vi "set transfer settings id.vi"(8 "error in (no error)":errorcluster, 9 "settings id":string, 10 "id":string, 11 "DSFConfiguration in":refnum<class "DSFConfiguration.lvclass">) -> (0 "error out":errorcluster, 3 "DSFConfiguration out":refnum<class "DSFConfiguration.lvclass">)   [LabVIEW 2017, in "DSFConfiguration.lvclass"]
uses:
  DSFConfiguration.lvclass
  DSFConfiguration.lvclass/DSFConfiguration.ctl
  DSFTransfer/DSFTransfer.lvclass/DSFTransfer.ctl
  DSFTransfer/Write settings id.vi
  DSFTransfer/DSFTransfer.lvclass
  C:/github/data-sharing-framework/Source/Configuration API/Classes/IDable/IDable.lvclass
  DSFPluginSettings/DSFPluginSettings.lvclass
  ID API/ID API.lvclass
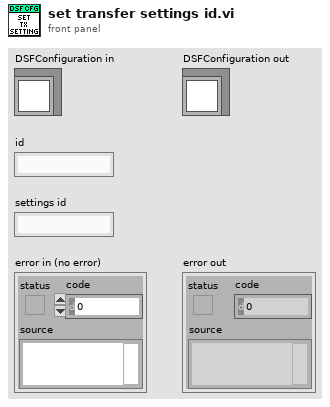
[diagram p1: front panel]
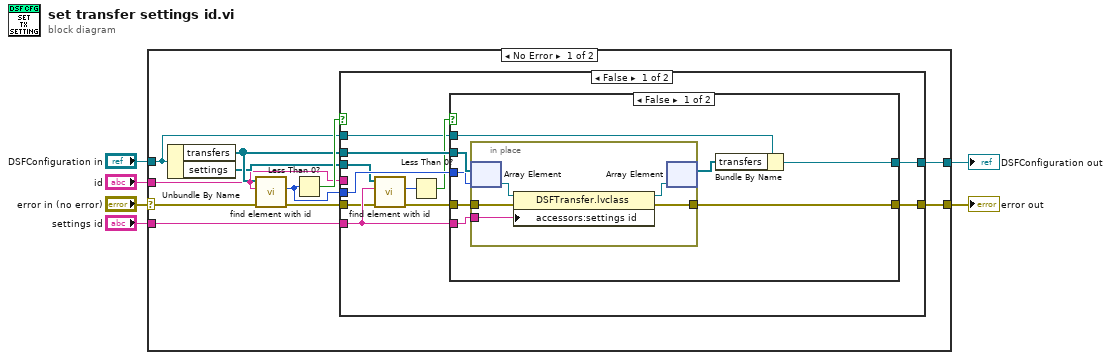
[diagram p0: block diagram]
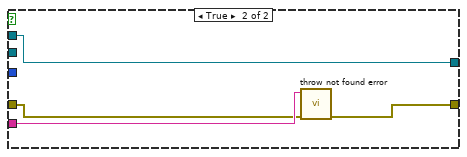
[diagram p2: hidden frame]
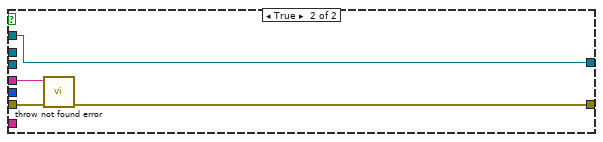
[diagram p3: hidden frame]
diagram:
  n1 = case shown="No Error" "error in (no error)" {
    selector: "error in (no error)" -> [w17 w51]
    tunnel: [w16 w51] -> w5
    tunnel: [w8 w50] -> w3
    tunnel: "DSFConfiguration in" -> [w9 w50]
    tunnel: "id" -> [w7 _]
    tunnel: "settings id" -> [w15 _]
    frame No Error {
      n2 = Unbundle By Name(w9) -> ("transfers"=w12:refnum<class "DSFTransfer.lvclass">[], "settings"=w10:refnum<class "DSFPluginSettings.lvclass">[])
      n3 = call "find element with id.vi"("error in (no error)"=w17, "id"=w7, "IDable Array in"=w12) -> ("error out"=w13:errorcluster, "index"=w11:i32)  [unwired: 7 in]
      n4 = Less Than 0?(x=w11) -> (x < 0?=w14:bool)
      n5 = case shown="False" w14 {
        tunnel: w13 -> [w19 w46]
        tunnel: [w26 w49] -> w16
        tunnel: w12 -> [w28 _]
        tunnel: w11 -> [w27 _]
        tunnel: w15 -> [w24 _]
        tunnel: [w25 w48] -> w8
        tunnel: w10 -> [w23 _]
        tunnel: w9 -> [w20 w48]
        tunnel: w7 -> [_ w47]
        frame False {
          n6 = call "find element with id.vi"("error in (no error)"=w19, "id"=w24, "IDable Array in"=w23) -> ("error out"=w18:errorcluster, "index"=w22:i32)  [unwired: 7 in]
          n7 = Less Than 0?(x=w22) -> (x < 0?=w21:bool)
          n8 = case shown="False" w21 {
            tunnel: w28 -> [w36 _]
            tunnel: w27 -> [w35 _]
            tunnel: w18 -> [w34 w42]
            tunnel: [w33 w45] -> w26
            tunnel: [w30 w44] -> w25
            tunnel: w24 -> [w32 w43]
            tunnel: w20 -> [w31 w44]
            frame False {
              n9 = in-place {
                in-place-border: w32 -> [w40]
                in-place-border: w34 -> [w38]
                in-place-border: [w37] -> w33
                n10 = in-place-array #1(w36, w35) -> (w41:refnum<class "DSFTransfer.lvclass">)
                n11 = property class="DSFTransfer.lvclass"(reference=w41, error in=w38, "accessors:settings id"=w40) -> (reference out=w39:refnum<class "DSFTransfer.lvclass">, error out=w37:errorcluster)
                n12 = in-place-array #1(w39) -> (w29:refnum<class "DSFTransfer.lvclass">[])  [unwired: 1 out]
              }
              n13 = Bundle By Name(cluster=w31, "transfers"=w29) -> (w30:refnum<class "DSFConfiguration.lvclass">)
            }
            frame True {
              n14 = call "throw not found error.vi"("error in (no error)"=w42, "id"=w43) -> ("error out"=w45:errorcluster)  [unwired: 9 in]
            }
          }
        }
        frame True {
          n15 = call "throw not found error.vi"("error in (no error)"=w46, "id"=w47) -> ("error out"=w49:errorcluster)  [unwired: 9 in]
        }
      }
    }
    frame Error {
    }
  }
  "error out" <- w5
  "DSFConfiguration out" <- w3
